vi "FL Create Variable.vi"(7 "name":string, 8 "error in (no error)":errorcluster, 9 "membership functions":T1[](array[typedef]) {"shape" items=["Triangle", "Trapezoid", "Singleton", "Sigmoid", "Gaussian", "User-Defined"]}, 10 "maximum":dbl=10.0, 11 "minimum":dbl=-10.0) -> (0 "error out":errorcluster, 3 "variable":T3 {"MFs"."shape" items=["Triangle", "Trapezoid", "Singleton", "Sigmoid", "Gaussian", "User-Defined"]})   [LabVIEW 2017, in "NI_Fuzzy_Logic_API.lvlib"]
doc: "Creates a linguistic variable for a fuzzy system. You also can use the <B>Variables</B> page of the Fuzzy System Designer to create linguistic variables interactively."
uses:
  <vilib>/addons/Fuzzy Logic/NI_Fuzzy_Logic_API.lvlib
  <vilib>/addons/Fuzzy Logic/TypeDefs/FL Variable.ctl
  <vilib>/addons/Fuzzy Logic/TypeDefs/FL Membership Function.ctl
  <vilib>/addons/Fuzzy Logic/TypeDefs/FL Membership Function Shape.ctl
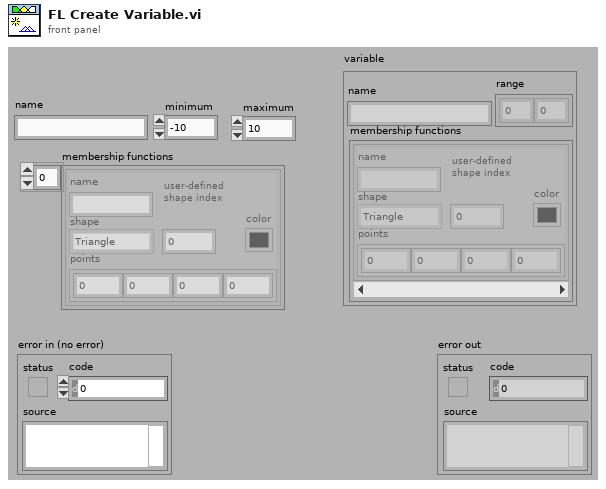
[diagram p1: front panel]
types:
  T1 = typedef "NI_Fuzzy_Logic_API.lvlib/FL Membership Function.ctl" = cluster{"name":string, "shape":T2, "points":dbl[], "color":u32, "user-defined shape index":i32}
  T2 = typedef "NI_Fuzzy_Logic_API.lvlib/FL Membership Function Shape.ctl" = u16
  T3 = typedef "NI_Fuzzy_Logic_API.lvlib/FL Variable.ctl" = cluster{"name":string, "range":dbl[], "MFs":T1[]}
  T4 = cluster{"Name":string, dbl[], "Membership Functions":T1[]}
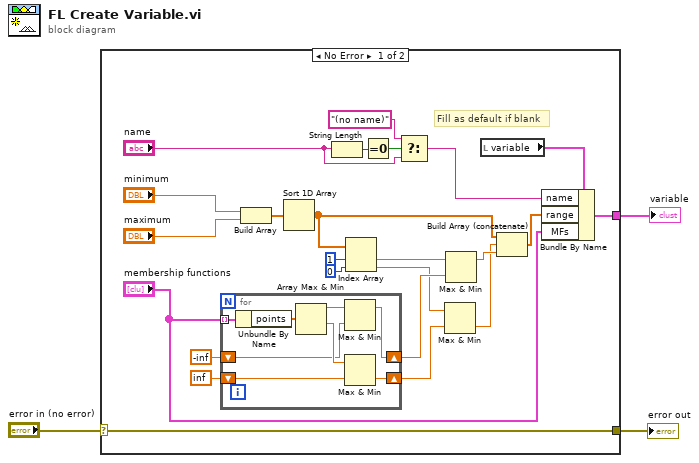
[diagram p0: block diagram]
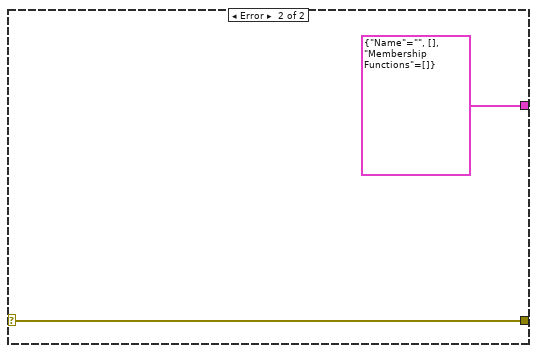
[diagram p2: hidden frame]
diagram:
  n1 = case shown="No Error" "error in (no error)" {
    selector: "error in (no error)" -> [w20 w37]
    tunnel: [w4 T4 {"Name"="", [], "Membership Functions"=[]}] -> w3
    tunnel: [w20 w37] -> w1
    frame No Error {
      # "Fill as default if blank"
      n2 = for {
        tunnel: "membership functions" -> [w35] mode=indexing
        shift-right: [w28] -> w14
        shift-left: -inf -> [w29]
        shift-right: [w31] -> w12
        shift-left: inf -> [w33]
        n3 = Unbundle By Name(w35) -> ("points"=w34:dbl[])
        n4 = Array Max & Min(array=w34) -> (max value=w30:dbl, min value=w32:dbl)  [unwired: 2 out]
        n5 = Max & Min(x=w30, y=w29) -> (max(x,y)=w28:dbl)  [unwired: 1 out]
        n6 = Max & Min(x=w32, y=w33) -> (min(x,y)=w31:dbl)  [unwired: 1 out]
      }
      n7 = Build Array("minimum", "maximum") -> (w21:dbl[])
      n8 = Sort 1D Array(array=w21) -> (sorted array=w9:dbl[])
      n9 = String Length(string="name") -> (length=w27:i32)
      n10 = Index Array(array=w9, index #1=1 ("index"), index #2=0 ("index")) -> (element #1=w15:dbl, element #2=w13:dbl)
      n11 = Equal To 0?(x=w27) -> (x = 0?=w26:bool)
      n12 = Select(t="(no name)", s=w26, f="name") -> (s? t:f=w7:string)
      n13 = Max & Min(x=w13, y=w12) -> (min(x,y)=w10:dbl)  [unwired: 1 out]
      n14 = Max & Min(x=w15, y=w14) -> (max(x,y)=w11:dbl)  [unwired: 1 out]
      n15 = local read "variable"() -> (w8:T3)
      n16 = Build Array (concatenate)(w9, w10, w11) -> (w6:dbl[])
      n17 = Bundle By Name(cluster=w8, "name"=w7, "range"=w6, "MFs"="membership functions") -> (w4:T3)
    }
    frame Error {
    }
  }
  "variable" <- w3
  "error out" <- w1
